vi "calculateTotalOfRobotModelTests.vi"(4 "Vf":dbl, 5 "fixed_V_sent?":bool=TRUE, 6 "V0":dbl, 7 "V_sent":dbl, 8 "error in (no error)":errorcluster, 9 "delta":dbl, 10 "quantity of samples":dbl, 11 "Game in":refnum<class "Game.lvclass">) -> (0 "error out":errorcluster, 1 "triples (V0, Vf, V_sent)":dbl[][](array[numeric]), 2 "totalNumerOfTests":dbl, 3 "Game out":refnum<class "Game.lvclass">)   [LabVIEW 2020, in "Game.lvclass"]
uses:
  Game.lvclass
  <vilib>/Analysis/1siggen.llb/Ramp Pattern by Delta.vi
  <vilib>/Analysis/NI_AALBase.lvlib
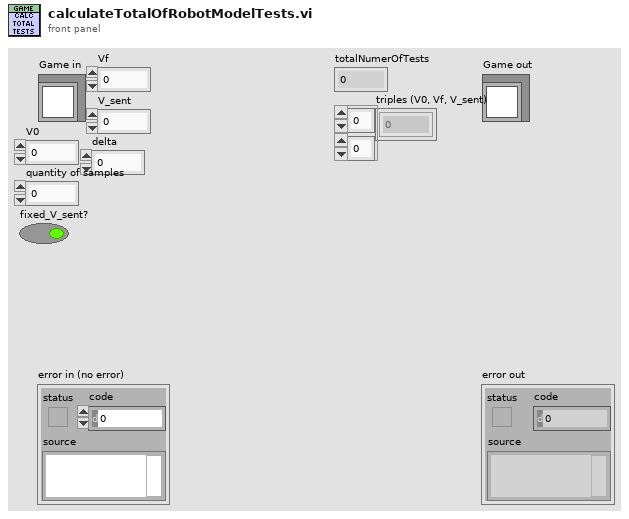
[diagram p1: front panel]
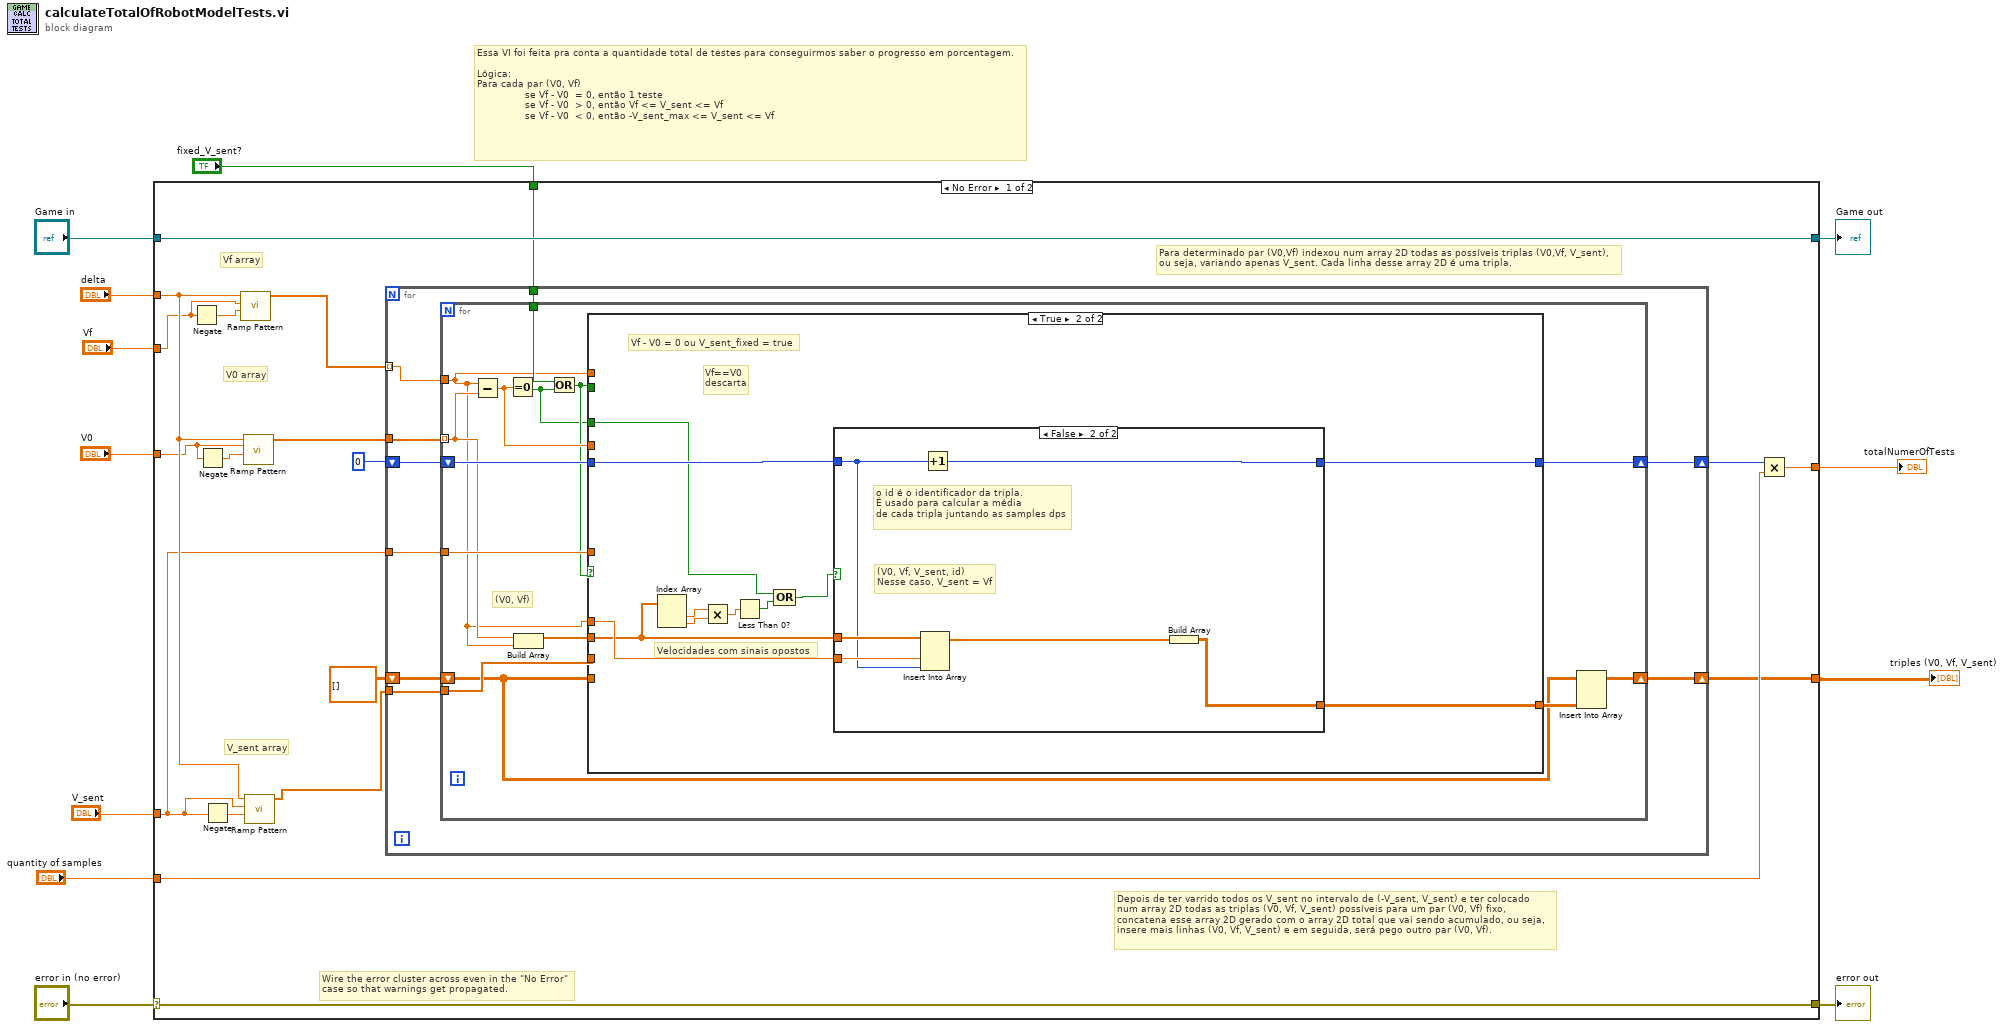
[diagram p0: block diagram]
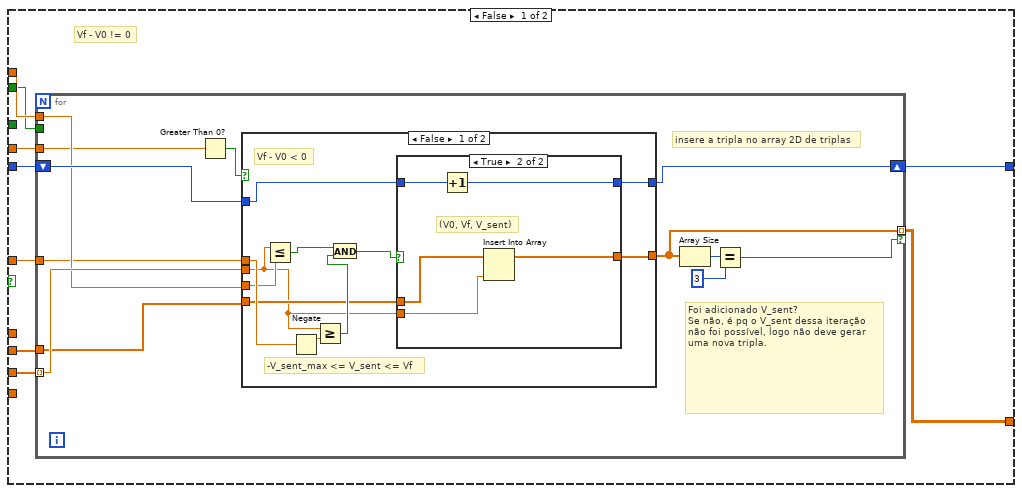
[diagram p2: hidden frame]
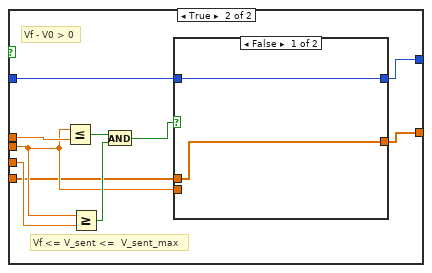
[diagram p4: hidden frame]
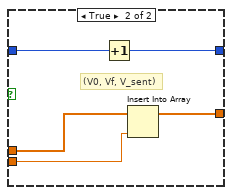
[diagram p5: hidden frame]
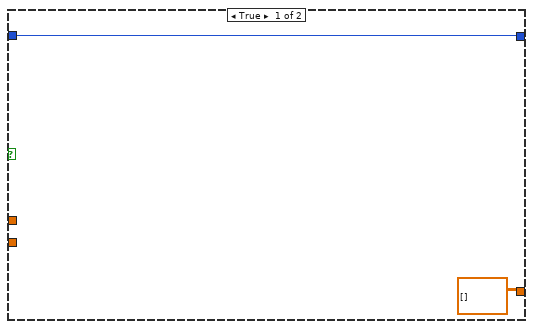
[diagram p6: hidden frame]
diagram:
  # "Essa VI foi feita pra conta a quantidade total de testes para conseguirmos saber o progresso em porcentagem.\n\nLógica:\nPara cada par (V0, Vf)\n                se Vf - V0  = 0, então 1 teste\n                se Vf - V0  > 0, então Vf <= V_sent <= Vf\n                se Vf - V0  < 0, então -V_sent_max <= V_sent <= Vf"
  n1 = case shown="No Error" "error in (no error)" {
    selector: "error in (no error)" -> [w30 w131]
    tunnel: [w30 w131] -> w11
    tunnel: [w31 w130] -> w9
    tunnel: "Game in" -> [w31 w130]
    tunnel: "delta" -> [w29 _]
    tunnel: "Vf" -> [w22 _]
    tunnel: "V0" -> [w13 _]
    tunnel: "V_sent" -> [w20 _]
    tunnel: [w24 _] -> w4
    tunnel: "quantity of samples" -> [w25 _]
    tunnel: "fixed_V_sent?" -> [w19 _]
    tunnel: [w18 _] -> w1
    frame No Error {
      # "Depois de ter varrido todos os V_sent no intervalo de (-V_sent, V_sent) e ter colocado\nnum array 2D todas as triplas (V0, Vf, V_sent) possíveis para um par (V0, Vf) fixo,\nconcatena esse array 2D gerado com o array 2D total que vai sendo acumulado, ou seja,\ninsere mais linhas (V0, Vf, V_sent) e em seguida, será pego outro par (V0, Vf)."
      # "Para determinado par (V0,Vf) indexou num array 2D todas as possíveis triplas (V0,Vf, V_sent),\nou seja, variando apenas V_sent. Cada linha desse array 2D é uma tripla."
      # "V_sent array"
      # "V0 array"
      # "Vf array"
      # "Wire the error cluster across even in the \"No Error\"\ncase so that warnings get propagated."
      n2 = Negate(x=w22) -> (-x=w23:dbl)
      n3 = Negate(x=w13) -> (-x=w14:dbl)
      n4 = Negate(x=w20) -> (-x=w21:dbl)
      n5 = call-poly <vilib>:"Ramp Pattern.vi"("start"=w23, "end"=w22, "delta"=w29) -> ("Ramp Pattern"=w16:dbl[])  [unwired: 6 in, 2 out]
      n6 = call-poly <vilib>:"Ramp Pattern.vi"("start"=w14, "end"=w13, "delta"=w29) -> ("Ramp Pattern"=w28:dbl[])  [unwired: 6 in, 2 out]
      n7 = call-poly <vilib>:"Ramp Pattern.vi"("start"=w21, "end"=w20, "delta"=w29) -> ("Ramp Pattern"=w15:dbl[])  [unwired: 6 in, 2 out]
      n8 = for {
        tunnel: w16 -> [w38] mode=indexing
        tunnel: w28 -> [w40]
        tunnel: w15 -> [w39]
        shift-right: [w37] -> w26
        shift-left: 0 -> [w36]
        tunnel: w20 -> [w35]
        tunnel: w19 -> [w34]
        shift-right: [w33] -> w18
        shift-left: dbl[][] [] -> [w32]
        n9 = for {
          tunnel: w40 -> [w48] mode=indexing
          tunnel: w39 -> [w46]
          tunnel: w38 -> [w41]
          shift-right: [w54] -> w37
          shift-left: w36 -> [w53]
          tunnel: w35 -> [w52]
          tunnel: w34 -> [w50]
          shift-right: [w43] -> w33
          shift-left: w32 -> [w44]
          # "(V0, Vf)"
          n10 = Subtract(x=w41, y=w48) -> (x-y=w51:dbl)
          n11 = Equal To 0?(x=w51) -> (x = 0?=w42:bool)
          n12 = Build Array(w48, w41) -> (w47:dbl[])
          n13 = Or(x=w50, y=w42) -> (x .or. y?=w49:bool)
          n14 = case shown="True" w49 {
            tunnel: w46 -> [w63 _]
            tunnel: w41 -> [w62 _]
            tunnel: [w61 w120] -> w54
            tunnel: w53 -> [w60 w121]
            tunnel: w52 -> [w59 _]
            tunnel: w49 -> [w58 _]
            tunnel: w51 -> [w57 _]
            tunnel: w41 -> [_ w119]
            tunnel: w47 -> [w56 w114]
            tunnel: [w55 w118] -> w45
            tunnel: w44 -> [_ _]
            tunnel: w42 -> [_ w113]
            frame False {
              # "Vf - V0 != 0"
              n15 = for {
                tunnel: w63 -> [w73] mode=indexing
                tunnel: w62 -> [w72]
                shift-right: [w74] -> w61
                shift-left: w60 -> [w75]
                tunnel: w59 -> [w71]
                tunnel: w58 -> [_]
                tunnel: w57 -> [w70]
                tunnel: w56 -> [w68]
                tunnel: [w65] -> w55 mode=indexing if=w64
                # "insere a tripla no array 2D de triplas"
                # "Foi adicionado V_sent?\nSe não, é pq o V_sent dessa iteração não foi possível, logo não deve gerar uma nova tripla."
                n16 = Greater Than 0?(x=w70) -> (x > 0?=w69:bool)
                n17 = case shown="False" w69 {
                  tunnel: w73 -> [w77 w96]
                  tunnel: w72 -> [w84 w102]
                  tunnel: w71 -> [w85 w100]
                  tunnel: w75 -> [w80 w98]
                  tunnel: [w79 w97] -> w74
                  tunnel: w68 -> [w78 w95]
                  tunnel: [w76 w94] -> w65
                  frame False {
                    # "-V_sent_max <= V_sent <= Vf"
                    # "Vf - V0 < 0"
                    n18 = Less Or Equal?(x=w77, y=w84) -> (x <= y?=w83:bool)
                    n19 = Negate(x=w85) -> (-x=w86:dbl)
                    n20 = Greater Or Equal?(x=w77, y=w86) -> (x >= y?=w82:bool)
                    n21 = And(x=w83, y=w82) -> (x .and. y?=w81:bool)
                    n22 = case shown="True" w81 {
                      tunnel: w80 -> [w87 w93]
                      tunnel: [w87 w92] -> w79
                      tunnel: w78 -> [w88 w91]
                      tunnel: w77 -> [_ w90]
                      tunnel: [w88 w89] -> w76
                      frame False {
                      }
                      frame True {
                        # "(V0, Vf, V_sent)"
                        n23 = Increment(x=w93) -> (x+1=w92:i32)
                        n24 = Insert Into Array(array=w91, new element=w90) -> (w89:dbl[])  [unwired: 1 in]
                      }
                    }
                  }
                  frame True {
                    # "Vf <= V_sent <=  V_sent_max"
                    # "Vf - V0 > 0"
                    n25 = Less Or Equal?(x=w96, y=w100) -> (x <= y?=w103:bool)
                    n26 = Greater Or Equal?(x=w96, y=w102) -> (x >= y?=w101:bool)
                    n27 = And(x=w103, y=w101) -> (x .and. y?=w99:bool)
                    n28 = case shown="False" w99 {
                      tunnel: w98 -> [w104 w110]
                      tunnel: [w104 w109] -> w97
                      tunnel: w96 -> [_ w108]
                      tunnel: w95 -> [w105 w107]
                      tunnel: [w105 w106] -> w94
                      frame False {
                      }
                      frame True {
                        # "(V0, Vf, V_sent)"
                        n29 = Increment(x=w110) -> (x+1=w109:i32)
                        n30 = Insert Into Array(array=w107, new element=w108) -> (w106:dbl[])  [unwired: 1 in]
                      }
                    }
                  }
                }
                n31 = Array Size(array=w65) -> (size(s)=w67:i32)
                n32 = Equal?(x=w67, y=3) -> (x = y?=w64:bool)
              }
            }
            frame True {
              # "Velocidades com sinais opostos"
              # "Vf==V0\ndescarta"
              # "Vf - V0 = 0 ou V_sent_fixed = true"
              n33 = Index Array(array=w114) -> (element #1=w116:dbl, element #2=w117:dbl)  [unwired: 2 in]
              n34 = Multiply(x=w116, y=w117) -> (x*y=w115:dbl)
              n35 = Less Than 0?(x=w115) -> (x < 0?=w112:bool)
              n36 = Compound Arithmetic op=OR(w113, w112) -> (w111:bool)
              n37 = case shown="False" w111 {
                tunnel: w121 -> [w123 w124]
                tunnel: [w123 w129] -> w120
                tunnel: w114 -> [_ w128]
                tunnel: w119 -> [_ w127]
                tunnel: [dbl[][] [] w125] -> w118
                frame True {
                }
                frame False {
                  # "o id é o identificador da tripla.\nÉ usado para calcular a média\nde cada tripla juntando as samples dps"
                  # "(V0, Vf, V_sent, id)\nNesse caso, V_sent = Vf"
                  n38 = Insert Into Array(array=w128, new element #1=w127, new element #2=w124) -> (w126:dbl[])  [unwired: 1 in]
                  n39 = Increment(x=w124) -> (x+1=w129:i32)
                  n40 = Build Array(w126) -> (w125:dbl[][])
                }
              }
            }
          }
          n41 = Insert Into Array(array=w44, new element=w45) -> (w43:dbl[][])  [unwired: 2 in]
        }
      }
      n42 = Multiply(x=w26, y=w25) -> (x*y=w24:dbl)
    }
    frame Error {
    }
  }
  "error out" <- w11
  "Game out" <- w9
  "totalNumerOfTests" <- w4
  "triples (V0, Vf, V_sent)" <- w1
